vi "Update Camera Modes.vi"(8 "error in (no error)":errorcluster, 10 "StringsAndValues":cluster{"String":string, "Value":i32}[](array[cluster]), 11 "Application in":refnum<class "Application.lvclass">) -> (0 "error out":errorcluster, 3 "Application out":refnum<class "Application.lvclass">)   [LabVIEW 2023, in "Application.lvlib" / "Application.lvclass"]
uses:
  Application.lvclass
  Application.lvclass/Application.ctl
  User Interface/Main Window Messages/Update Camera Modes Msg/Update Camera Modes Msg.lvclass/Update Camera Modes Msg.ctl
  <vilib>/ActorFramework/Message Enqueuer/Message Enqueuer.lvclass/Message Enqueuer.ctl
  <vilib>/ActorFramework/Message Enqueuer/Enqueue.vi
  User Interface/Main Window Messages/Update Camera Modes Msg/Update Camera Modes Msg.lvclass
  C:/Program Files/National Instruments/LabVIEW 2023/vi.lib/ActorFramework/Message/Message.lvclass
  <vilib>/ActorFramework/Message Priority Queue/Priority Enqueue.vi
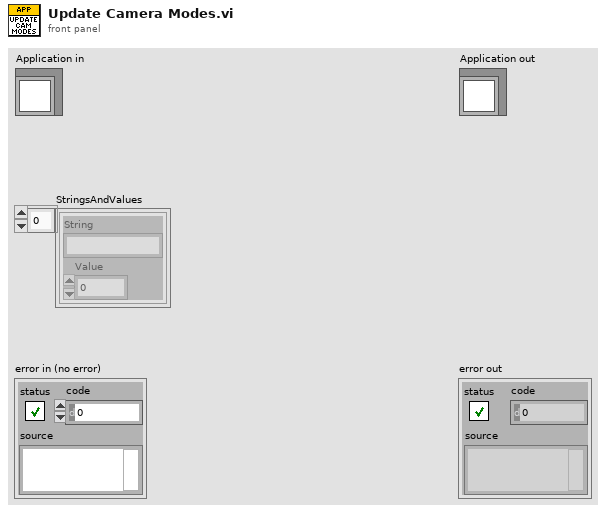
[diagram p1: front panel]
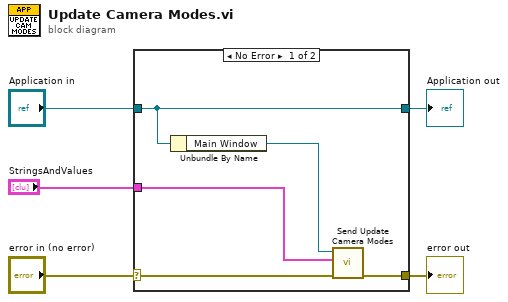
[diagram p0: block diagram]
diagram:
  n1 = case shown="No Error" "error in (no error)" {
    selector: "error in (no error)" -> [w9 w12]
    tunnel: [w8 w12] -> w4
    tunnel: [w10 w11] -> w2
    tunnel: "Application in" -> [w10 w11]
    tunnel: "StringsAndValues" -> [w6 _]
    frame No Error {
      n2 = Unbundle By Name(w10) -> ("Main Window"=w7:refnum<class "Message Enqueuer.lvclass">)
      n3 = call "Send Update Camera Modes.vi"("error in (no error)"=w9, "StringsAndValues"=w6, "Message Enqueuer"=w7) -> ("error out"=w8:errorcluster)  [unwired: 7 in, 1 out]
    }
    frame Error {
    }
  }
  "error out" <- w4
  "Application out" <- w2
